vi "Write_to_Database.vi"(2 "Database name":string, 3 "Detector ID":i32, 4 "Error in":errorcluster, 5 "Message status ID":string, 6 "Weather Parameter String":string, 7 "Message type ID":string) -> (0 "Error out":errorcluster, 1 "Data Buffer?":bool)   [LabVIEW 2013]
uses:
  <vilib>/addons/database/Connection.llb/DB Tools Open Connec (String).vi
  <vilib>/addons/database/NI_Database_API.lvlib
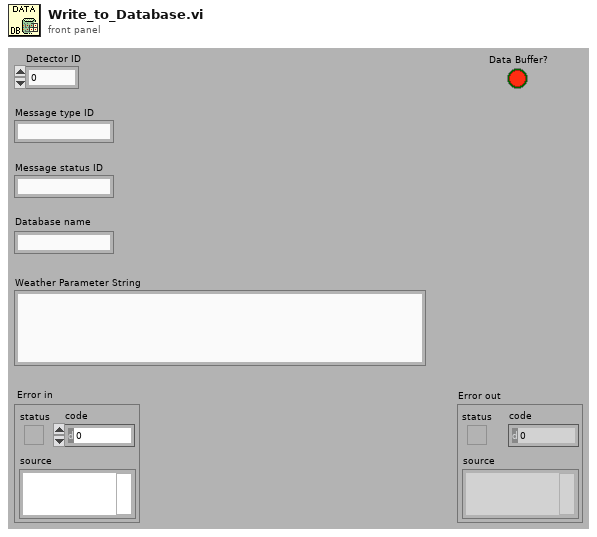
[diagram p1: front panel]
types:
  T1 = typedef "NI_Database_API.lvlib/Conn ObjectReference.ctl" = refnum<k1>
  T2 = cluster{"Detector ID":i32, "Message type ID":string, "Message status ID":string, "Weather Parameter String":string}
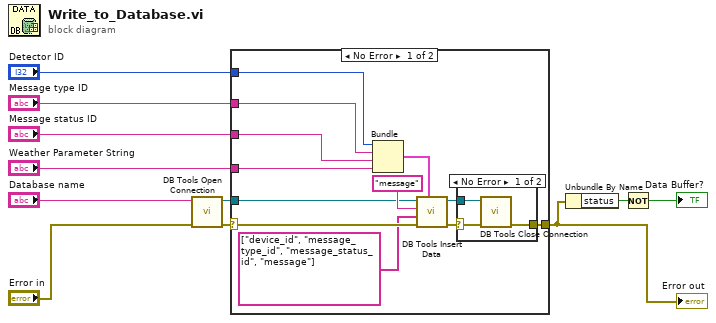
[diagram p0: block diagram]
diagram:
  n1 = call-poly <vilib>:"DB Tools Open Connection.vi"("error in (no error)"="Error in", "connection information"="Database name") -> ("error out"=w6:errorcluster, "connection reference"=w7:T1)  [unwired: 6 in]
  n2 = case shown="No Error" w6 {
    selector: w6 -> [w17 w28]
    tunnel: "Weather Parameter String" -> [w20 _]
    tunnel: "Detector ID" -> [w19 _]
    tunnel: w7 -> [w18 _]
    tunnel: [w14 w28] -> w5
    tunnel: "Message type ID" -> [w13 _]
    tunnel: "Message status ID" -> [w12 _]
    frame No Error {
      n3 = Bundle("Detector ID"=w19, "Message type ID"=w13, "Message status ID"=w12, "Weather Parameter String"=w20) -> (w22:T2)  [unwired: 1 out]
      n4 = call <vilib>:"DB Tools Insert Data.vi"("data"=w22, "error in (no error)"=w17, "columns"=string[] ["device_id", "message_type_id", "message_status_id", "message"], "table"="message", "connection reference"=w18) -> ("error out"=w15:errorcluster, "connection reference out"=w23:T1)  [unwired: 2 in, 3 out]
      n5 = case shown="No Error" w15 {
        selector: w15 -> [w25 w27]
        tunnel: w23 -> [w26 _]
        tunnel: [w24 w27] -> w14
        frame No Error {
          n6 = call <vilib>:"DB Tools Close Connection.vi"("error in (no error)"=w25, "connection reference"=w26) -> ("error out"=w24:errorcluster)  [unwired: 5 in]
        }
        frame Error {
        }
      }
    }
    frame Error {
    }
  }
  "Error out" <- w5
  n7 = Unbundle By Name(w5) -> ("status"=w4:bool)
  n8 = Not(x=w4) -> (.not. x?=→"Data Buffer?":bool)
